vi "Generic Request (Buffer).vi"(5 "method":string, 6 "timeout":i32=10000, 7 "output file":path, 8 "error in":errorcluster, 9 "buffer":string, 10 "url":string, 11 "Session In":refnum<class "Session.lvclass">) -> (0 "error out":errorcluster, 1 "body":string, 2 "headers":string, 3 "Session Out":refnum<class "Session.lvclass">, 4 "status code":u32)   [LabVIEW 2020, in "Library Commun.lvlib" / "Library Http.lvlib" / "Session.lvclass"]
uses:
  Session.lvclass
  Session.lvclass/Session.ctl
  lvwebclient_32.dll
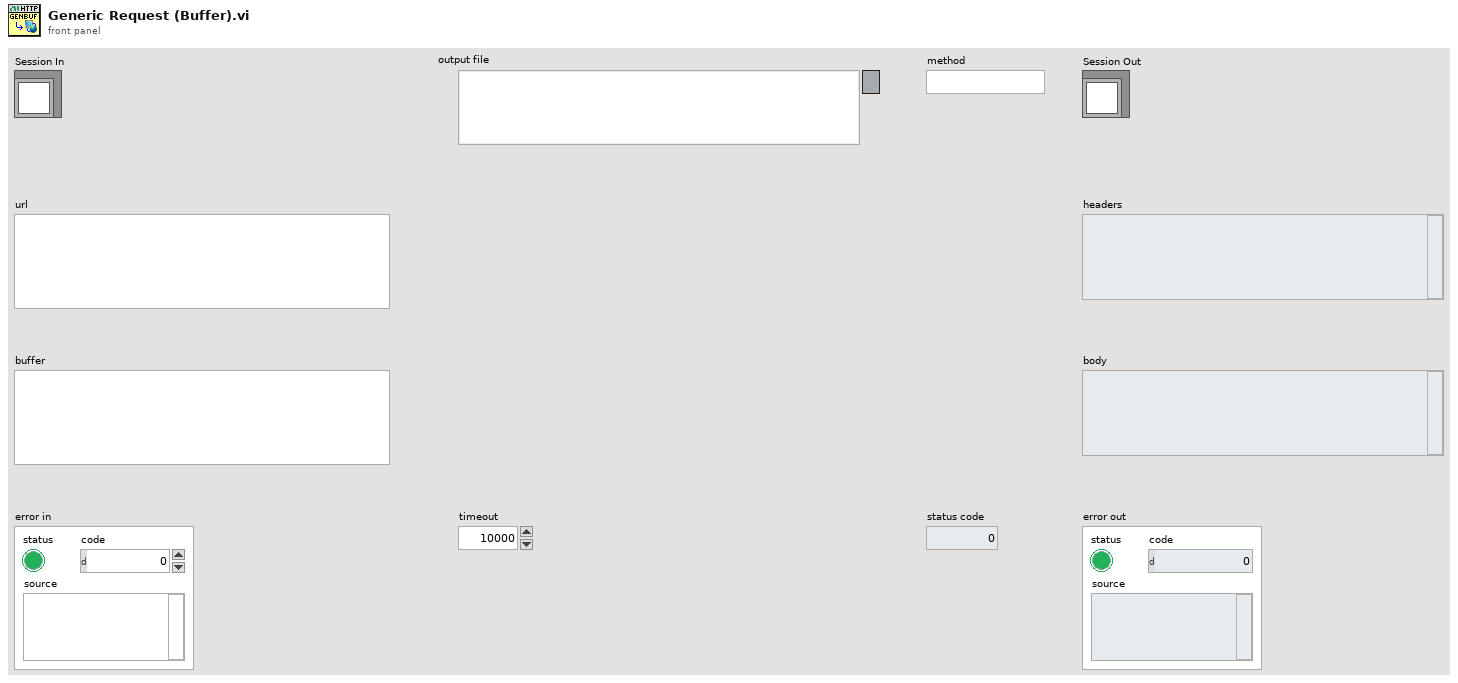
[diagram p1: front panel]
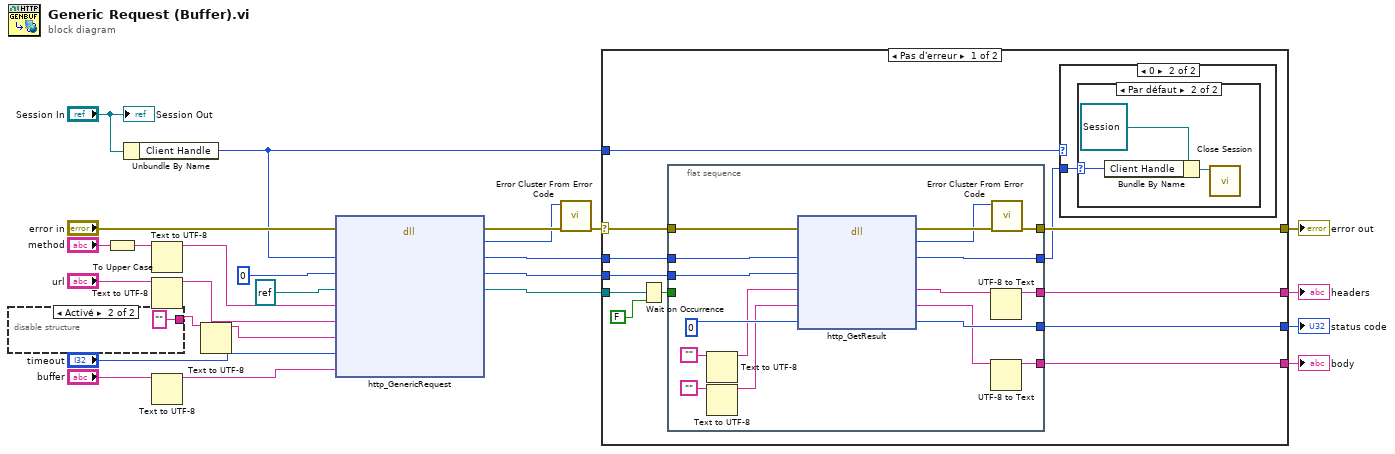
[diagram p0: block diagram]
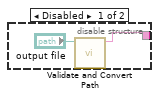
[diagram p2: hidden frame]
diagram:
  n1 = disable-structure shown="Activé" {
    disable-tunnel: [w26 "" ("validated path as string")] -> w2
    frame Disabled {
      n2 = call "Validate and Convert Path.vi"("path"="output file") -> ("validated path as string"=w26:string)  [unwired: 10 in]
    }
    frame Enabled {
    }
  }
  n3 = To Upper Case(1:"method") -> (0:w3:string)
  n4 = Unbundle By Name("Session In") -> ("Client Handle"=w9:u32)
  n5 = Text to UTF-8(11:w3) -> (3:w6:string)  [unwired: 2 in, 1 out]
  n6 = Text to UTF-8(11:"url") -> (3:w8:string)  [unwired: 2 in, 1 out]
  n7 = Text to UTF-8(11:"buffer") -> (3:w4:string)  [unwired: 2 in, 1 out]
  n8 = Text to UTF-8(11:w2) -> (3:w1:string)  [unwired: 2 in, 1 out]
  n9 = dll-call lib="C:/Users/ngarcin/OneDrive - Altyor/Standard TB/Class/Http Altyor/lvwebclient_*.*" fn="http_GenericRequest"(error in="error in", "handle"=w9, "request"=u32 0, "completeOccurrence"=refnum<k4> refnum ("occurrence"), "method"=w6, "url"=w8, "outPath"=w1, "timeoutInMs"="timeout", "requestBody"=w4) -> (error out=w17:errorcluster, "return"=w16:i32, "handle"=w15:u32, "request"=w14:u32, "completeOccurrence"=w12:refnum<k4>)  [unwired: 7 in, 1 out]
  n10 = call <vilib>:"Error Cluster From Error Code.vi"("error in (no error)"=w17, "error code (0)"=w16) -> ("error out"=w25:errorcluster)  [unwired: 7 in]
  n11 = case shown="Pas d'erreur" w25 {
    selector: w25 -> [w38 w62]
    tunnel: w12 -> [w40 _]
    tunnel: w15 -> [w37 _]
    tunnel: w14 -> [w36 _]
    tunnel: [w35 _] -> w22
    tunnel: [w34 _] -> w21
    tunnel: [w33 _] -> w20
    tunnel: [w32 w62] -> w19
    tunnel: w9 -> [w31 _]
    frame No Error {
      n12 = Wait on Occurrence(1:FALSE, 2:w40) -> (0:w39:bool)  [unwired: 1 in]
      n13 = flat-sequence {
        tunnel: w39 -> [_]
        tunnel: w38 -> [w61]
        tunnel: w37 -> [w60]
        tunnel: w36 -> [w59]
        tunnel: [w57] -> w35
        tunnel: [w52] -> w34
        tunnel: [w51] -> w33
        tunnel: [w50] -> w32
        tunnel: [w49] -> w30
        frame #0 {
          n14 = Text to UTF-8(11:"") -> (3:w46:string)  [unwired: 2 in, 1 out]
          n15 = Text to UTF-8(11:"") -> (3:w45:string)  [unwired: 2 in, 1 out]
          n16 = dll-call lib="C:/Users/ngarcin/OneDrive - Altyor/Standard TB/Class/Http Altyor/lvwebclient_*.*" fn="http_GetResult"(error in=w61, "handle"=w60, "request"=w59, "returnHeader"=w46, "returnBody"=w45, "httpStatus"=u32 0) -> (error out=w56:errorcluster, "return"=w55:i32, "handle"=w49:u32, "returnHeader"=w54:string, "returnBody"=w53:string, "httpStatus"=w57:u32)  [unwired: 3 in, 1 out]
          n17 = UTF-8 to Text(11:w54) -> (3:w52:string)  [unwired: 2 in, 1 out]
          n18 = UTF-8 to Text(11:w53) -> (3:w51:string)  [unwired: 2 in, 1 out]
          n19 = call <vilib>:"Error Cluster From Error Code.vi"("error in (no error)"=w56, "error code (0)"=w55) -> ("error out"=w50:errorcluster)  [unwired: 7 in]
        }
      }
      n20 = case shown="0" w31 {
        tunnel: w30 -> [_ w41]
        frame Default {
        }
        frame 0 {
          n21 = case shown="Par défaut" w41 {
            selector: w41 -> [_ w44]
            frame 0 {
            }
            frame Default {
              n22 = Bundle By Name(cluster=refnum<class "Session.lvclass"> refnum ("Session Out"), "Client Handle"=w44) -> (w42:refnum<class "Session.lvclass">)
              n23 = call "Close Session.vi"("Session In"=w42) -> ()  [unwired: 10 in, 1 out]
            }
          }
        }
      }
    }
    frame Error {
    }
  }
  "error out" <- w19
  "headers" <- w21
  "body" <- w20
  "status code" <- w22
  "Session Out" <- "Session In"
